vi "FPGA_Main_R2.vi"() -> ()   [LabVIEW 2018]
uses:
  <userlib>/_NI I2C IP/FPGA/Public/Data Array Type.ctl
  Data Def/FPGA_Digital Output.ctl
  Data Def/FPGA_Digital Input.ctl
  <userlib>/_NI I2C IP/FPGA/Public/I2C Interface.ctl
  <userlib>/_NI I2C IP/FPGA/Public/Word Controller Settings.ctl
  <vilib>/rvi/Emulation/niFpgaGetClockAttributes.vi
  <vilib>/rvi/Emulation/niFpgaSctlEmulationGetInTimedLoop.vi
  <vilib>/rvi/Emulation/niFpgaEmulationReportErrorSimple.vi
  <vilib>/rvi/eio/common/nirviEmuTemplateMethod_errors.vi
  <vilib>/rvi/interface/RandomDataEmulation/niFpgaRandomDataHandleErrors.vi
  <vilib>/rvi/Emulation/niFpgaCriticalErrorInLSC.vi
  <vilib>/eio/EIONode/EIONode.xnode
  <vilib>/rvi/DataTransferAndStorage/Container/XNode/niFpgaContainer.xnode
  <vilib>/rvi/interface/RandomDataEmulation/nirviRandomDataFpgaReadWriteTemplate.vi
  <vilib>/eio/EIOMethodNode/EIOMethodNode.xnode
  <userlib>/_NI I2C IP/FPGA/NI I2C IP FPGA.lvlib
panel:
  out "Overflow?":bool
  in  "DMA Write":bool
  out "read data":T1 format="%.0x"
  in  "Divide":u8
  in  "10-bit Addressing":bool
  in  "Number of Bytes":u8
  in  "Read":bool
  in  "Device Address":u16
  out "Ready for Input":bool
  in  "Write Data":T1=[0, 0, 0, 0, 0, 0, 0, 0] format="%.0x"
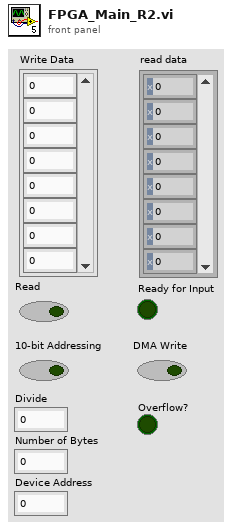
[diagram p1: front panel]
types:
  T1 = typedef "NI I2C IP FPGA.lvlib/Data Array Type.ctl" = u8[]
  T2 = typedef "FPGA_Digital Input.ctl" = cluster{"DI 0":refnum<k21>, "DI 1":refnum<k21>, "DI 2":refnum<k21>, "DI 3":refnum<k21>, "DI 4":refnum<k21>, "DI 5":refnum<k21>, "DI 6":refnum<k21>, "DI 7":refnum<k21>, "DI 8":refnum<k21>, "DI 9":refnum<k21>, "DI 10":refnum<k21>, "DI 11":refnum<k21>}
  T3 = typedef "FPGA_Digital Output.ctl" = cluster{"DO 0":refnum<k21>, "DO 1":refnum<k21>, "DO 2":refnum<k21>, "DO 3":refnum<k21>, "DO 4":refnum<k21>, "DO 5":refnum<k21>, "DO 6":refnum<k21>, "DO 7":refnum<k21>, "DO 8":refnum<k21>, "DO 9":refnum<k21>, "DO 10":refnum<k21>, "DO 11":refnum<k21>}
  T4 = typedef "NI I2C IP FPGA.lvlib/Word Controller Settings.ctl" = cluster{"Device Address":u16, "Read":bool, "Number of Bytes":u8, "10-bit Addressing":bool, "Divide":u8}
  T5 = typedef "NI I2C IP FPGA.lvlib/I2C Interface.ctl" = cluster{"Clock":bool, "Data":bool}
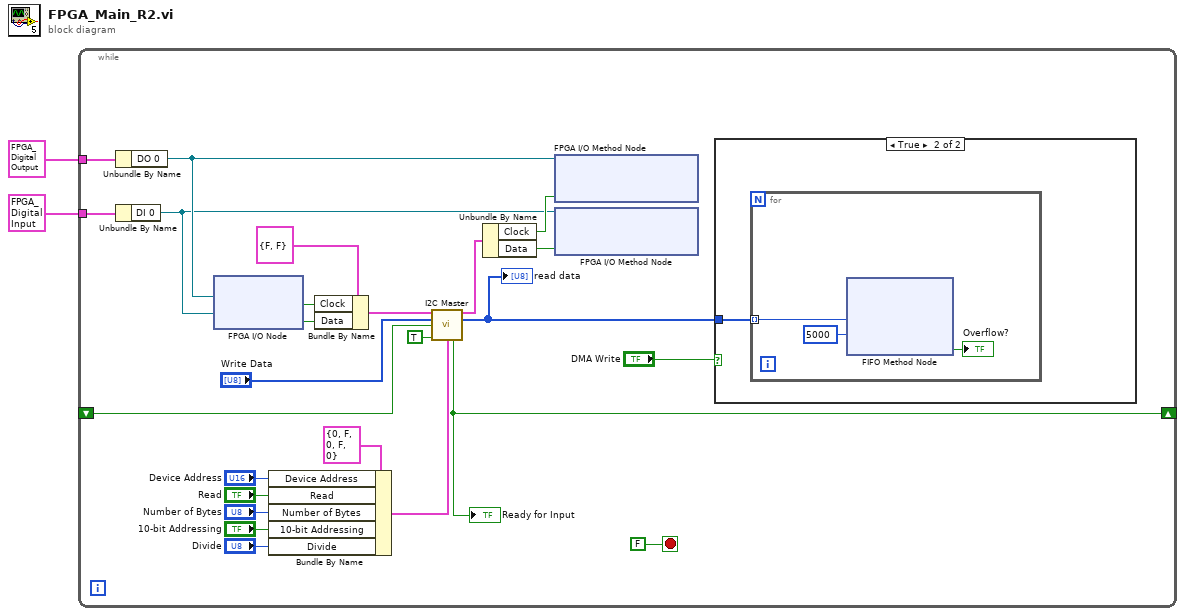
[diagram p0: block diagram]
diagram:
  n1 = while {
    tunnel: T3 {"DO 0"="RMC/DIO62", "DO 1"="RMC/DIO44", "DO 2"="RMC/DIO77", "DO 3"="RMC/DIO61", "DO 4"="RMC/DIO94", "DO 5"="RMC/DIO12", "DO 6"="RMC/DIO76", "DO 7"="RMC/DIO29", "DO 8"="RMC/DIO93", "DO 9"="RMC/DIO11", "DO 10"="RMC/DIO43", "DO 11"="RMC/DIO28"} ("Digital Output") -> [w27]
    tunnel: T2 {"DI 0"="RMC/DIO15", "DI 1"="RMC/DIO47", "DI 2"="RMC/DIO46", "DI 3"="RMC/DIO79", "DI 4"="RMC/DIO63", "DI 5"="RMC/DIO14", "DI 6"="RMC/DIO78", "DI 7"="RMC/DIO31", "DI 8"="RMC/DIO95", "DI 9"="RMC/DIO13", "DI 10"="RMC/DIO45", "DI 11"="RMC/DIO30"} ("Digital Input") -> [w26]
    shift-right: [w19] -> _
    shift-left: _ -> [w18]
    stop <- FALSE stop-if-true
    n2 = Unbundle By Name(w27) -> ("DO 0"=w8:refnum<k21>)
    n3 = Unbundle By Name(w26) -> ("DI 0"=w6:refnum<k21>)
    n4 = xnode "FPGA I/O Node"("FPGA I/O In"=w8, "FPGA I/O In"=w6) -> ("I/O Item"=w24:bool, "I/O Item"=w23:bool)  [unwired: 2 out]
    n5 = Bundle By Name(cluster=T4 {"Device Address"=0, "Read"=FALSE, "Number of Bytes"=0, "10-bit Addressing"=FALSE, "Divide"=0} ("settings"), "Device Address"="Device Address", "Read"="Read", "Number of Bytes"="Number of Bytes", "10-bit Addressing"="10-bit Addressing", "Divide"="Divide") -> (w11:T4)
    n6 = Bundle By Name(cluster=T5 {"Clock"=FALSE, "Data"=FALSE} ("i2c bus in"), "Clock"=w24, "Data"=w23) -> (w22:T5)
    n7 = call <userlib>:"I2C Master.vi"("i2c bus in"=w22, "write data"="Write Data", "go"=w18, "direction ready"=TRUE, "settings"=w11) -> ("i2c bus out"=w9:T5, "read data"=w4:T1, "ready for input"=w19:bool)  [unwired: 8 in]
    "Ready for Input" <- w19
    "read data" <- w4
    n8 = Unbundle By Name(w9) -> ("Clock"=w7:bool, "Data"=w5:bool)
    n9 = xnode "FPGA I/O Method Node"("FPGA I/O In"=w8, "Enable"=w7) -> ()  [unwired: 1 out]
    n10 = xnode "FPGA I/O Method Node"("FPGA I/O In"=w6, "Enable"=w5) -> ()  [unwired: 1 out]
    n11 = case shown="True" "DMA Write" {
      tunnel: w4 -> [_ w28]
      frame False {
      }
      frame True {
        n12 = for {
          tunnel: w28 -> [w31] mode=indexing
          n13 = xnode ("FIFO Method Node")("Element"=w31, "Timeout"=5000) -> ("Timed Out?"=→"Overflow?":bool)  [unwired: 1 in, 1 out]
        }
      }
    }
  }
